vi "Convert filetype to Is library type.vi"(4 "file type":T1) -> (1 "Is library type?":bool)   [LabVIEW 2020, in "NI_FileType.lvlib"]
doc: "Returns TRUE if this file type is a type of library, such as Libraries, XControls, XNodes, and LVClasses."
uses:
  NI_FileType.lvlib
  FT_FileTypes.ctl
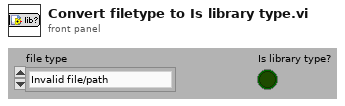
[diagram p1: front panel]
types:
  T1 = typedef "NI_FileType.lvlib/FT_FileTypes.ctl" = enum32{"Invalid file/path", "Unknown type", "Instrument", "Control", "Polymorphic VI", "Project", "Library", "LVClass", "XControl", "XNode", "CIN", "Run-time menu", "Palette menu", "LLB", "Shortcut", "Directory", "Class Private Data Control", "Statechart", "MathScript .m file", "Ladder Diagram", "LVLibp"}
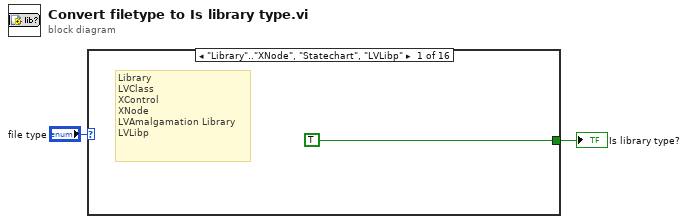
[diagram p0: block diagram]
diagram:
  n1 = case shown="\"Library\"..\"XNode\", \"Statechart\", \"LVLibp\"" "file type" {
    tunnel: [TRUE _ _ _ _ _ _ _ _ _ _ _ _ _ _ _] -> w2
    frame "Library".."XNode", "Statechart", "LVLibp" {
      # "Library\nLVClass\nXControl\nXNode\nLVAmalgamation Library\nLVLibp"
    }
    frame "CIN" {
    }
    frame "Run-time menu" {
    }
    frame "Palette menu" {
    }
    frame "LLB" {
    }
    frame "Shortcut" {
    }
    frame "Directory" {
    }
    frame "Class Private Data Control" {
    }
    frame "Project" {
    }
    frame "Polymorphic VI" {
    }
    frame "Control" {
    }
    frame "Instrument" {
    }
    frame "Unknown type" {
    }
    frame "Invalid file/path" {
    }
    frame "MathScript .m file" {
    }
    frame "Ladder Diagram" {
    }
  }
  "Is library type?" <- w2
